vi "MTUChipCornerSample.vi"() -> ()   [LabVIEW 2017, in "AOILib_MTUchipcorner_V1.lvlib"]
uses:
  <userlib>/AOILib_MTUchipcorner_V1/AOILib_MTUchipcorner_V1.lvlib
  <vilib>/vision/NI_Vision_Development_Module.lvlib
panel:
  in  "File Path_IMGin":path=path "C:/Users/MyUser/Desktop/Harvie Test/CornerChip/ChipCornerTest.bmp"
  out "image":T1(plugin-control)
  out "X Resolution":i32
  out "Y Resolution":i32
  in  "imageParm 2":T2={"PICmode"=0, "Outputmode"=0, "cols"=2448, "rows"=2048, "correctTheta"=0.0}
  in  "Param":T3={"Select Mode \n0: Dark\n1: light"=1.0, "Threshold Value"=200.0, "Chip Long Side Size"=25.0, "Chip Long Side Min Tolerance"=0.8, "Chip Long Side Max Tolerance"=1.5, "Chip Short Side Size"=15.0, "Chip Short Side Min Tolerance"=0.8, "Chip Short Side Max Tolerance"=1.5, "Chip Pitch X"=70.0, "Chip Pitch Y"=70.0, "Edge Exclusion Distance"=200.0, "Reserve[11]"=0.0, "Reserve[12]"=0.0, "Parameters[13]"=0.0, "Parameters[14]"=0.0, "Parameters[15]"=0.0, "Parameters[16]"=0.0, "Parameters[17]"=0.0, "Parameters[18]"=0.0, "Parameters[19]"=0.0}
  out "image out":T1(plugin-control)
  out "error out":errorcluster
  out "fAngle":sgl[](array[numeric])
  out "fPosY":sgl[](array[numeric])
  out "fPosX":sgl[](array[numeric])
  out "boolResult":sgl[](array[numeric])
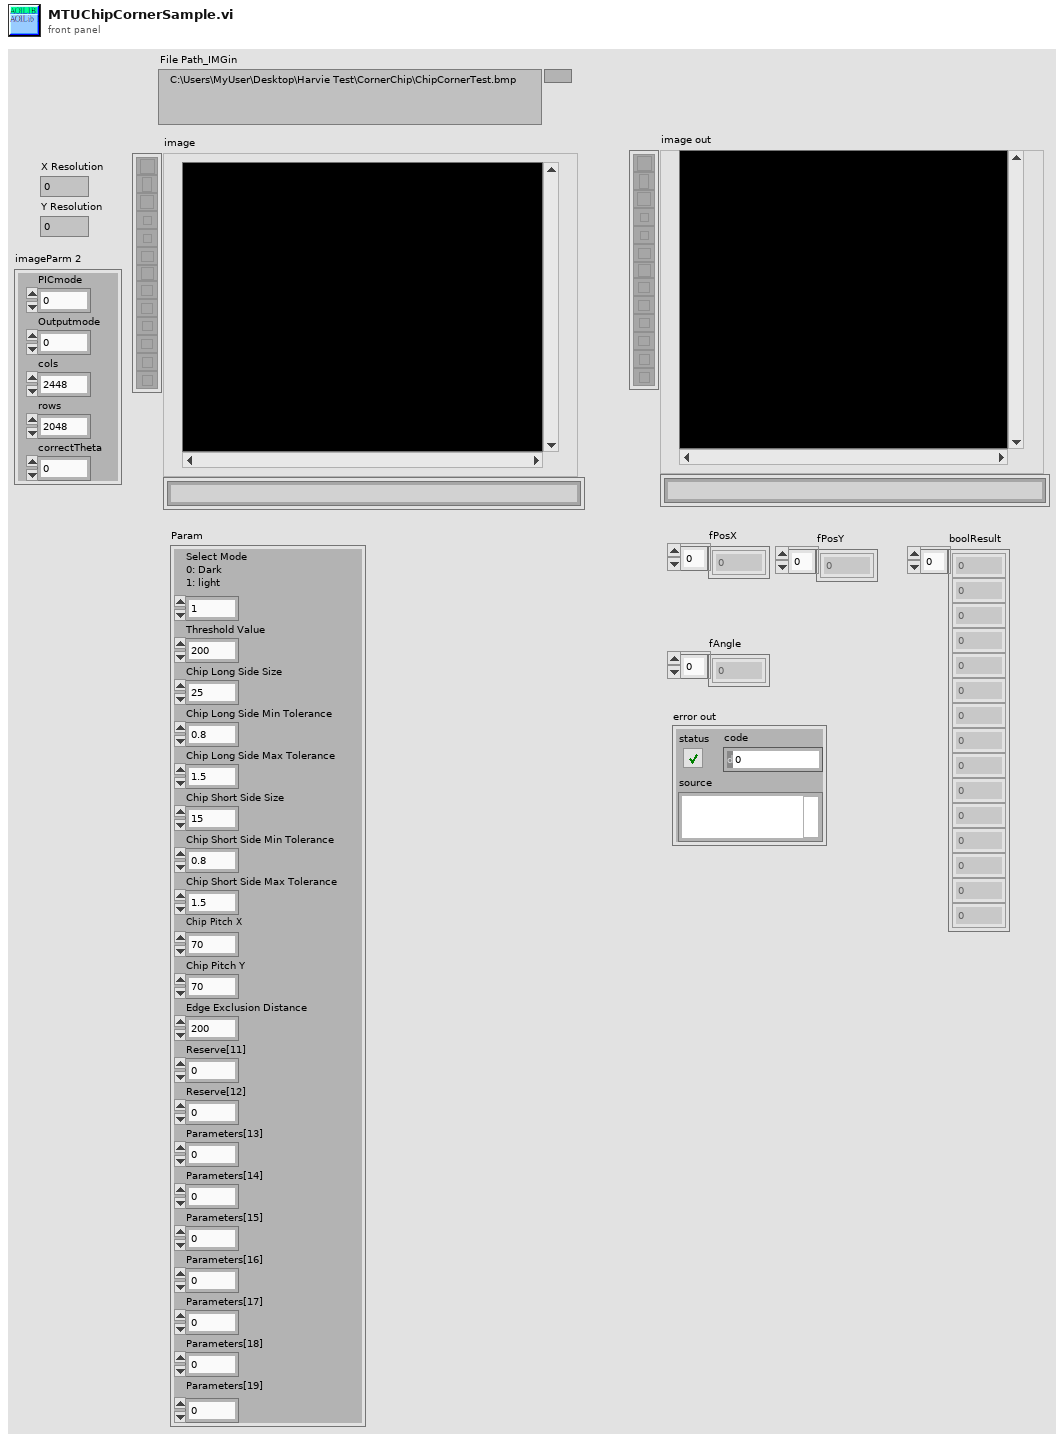
[diagram p1: front panel]
types:
  T1 = typedef "IMAQ Image.ctl" = refnum<image>
  T2 = cluster{"PICmode":i32, "Outputmode":i32, "cols":i32, "rows":i32, "correctTheta":dbl}
  T3 = cluster{"Select Mode \n0: Dark\n1: light":sgl, "Threshold Value":sgl, "Chip Long Side Size":sgl, "Chip Long Side Min Tolerance":sgl, "Chip Long Side Max Tolerance":sgl, "Chip Short Side Size":sgl, "Chip Short Side Min Tolerance":sgl, "Chip Short Side Max Tolerance":sgl, "Chip Pitch X":sgl, "Chip Pitch Y":sgl, "Edge Exclusion Distance":sgl, "Reserve[11]":sgl, "Reserve[12]":sgl, "Parameters[13]":sgl, "Parameters[14]":sgl, "Parameters[15]":sgl, "Parameters[16]":sgl, "Parameters[17]":sgl, "Parameters[18]":sgl, "Parameters[19]":sgl}
  T4 = typedef "Image Type" = u32
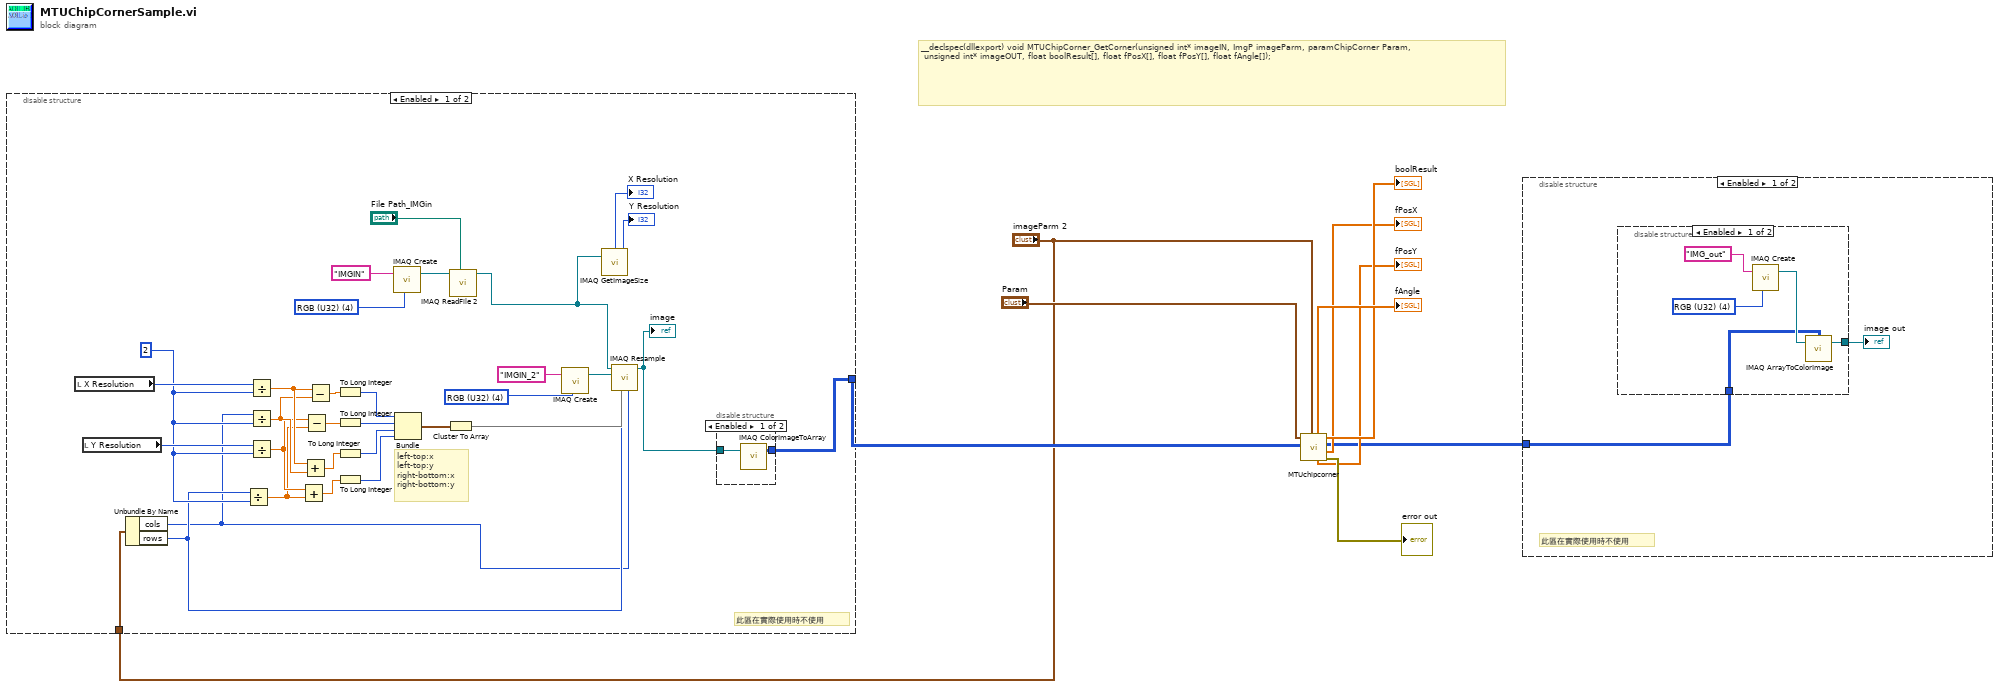
[diagram p0: block diagram]
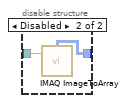
[diagram p2: hidden frame]
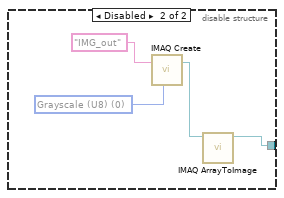
[diagram p4: hidden frame]
diagram:
  # "__declspec(dllexport) void MTUChipCorner_GetCorner(unsigned int* imageIN, ImgP imageParm, paramChipCorner Param,\n\tunsigned int* imageOUT, float boolResult[], float fPosX[], float fPosY[], float fAngle[]);"
  n1 = disable-structure shown="Enabled" {
    disable-tunnel: [w14 _] -> w2
    disable-tunnel: "imageParm 2" -> [w12 _]
    frame Enabled {
      w16 = T4 4 items=["Grayscale (U8)", "Grayscale (I16)", "Grayscale (SGL)", "Complex (CSG)", "RGB (U32)", "HSL (U32)", "RGB (U64)", "Grayscale (U16)"] ("Image Type")
      w17 = T4 4 items=["Grayscale (U8)", "Grayscale (I16)", "Grayscale (SGL)", "Complex (CSG)", "RGB (U32)", "HSL (U32)", "RGB (U64)", "Grayscale (U16)"] ("Image Type")
      w32 = 2 ("y")
      # "此區在實際使用時不使用"
      # "left-top:x\nleft-top:y\nright-bottom:x\nright-bottom:y"
      n2 = local read "X Resolution"() -> (w34:i32)
      n3 = local read "Y Resolution"() -> (w33:i32)
      n4 = Unbundle By Name(w12) -> ("cols"=w10:i32, "rows"=w11:i32)
      n5 = Divide(x=w11, y=w32) -> (x/y=w25:dbl)
      n6 = Divide(x=w34, y=w32) -> (x/y=w29:dbl)
      n7 = Divide(x=w10, y=w32) -> (x/y=w28:dbl)
      n8 = Divide(x=w33, y=w32) -> (x/y=w26:dbl)
      n9 = Add(x=w26, y=w25) -> (x+y=w24:dbl)
      n10 = Add(x=w29, y=w28) -> (x+y=w27:dbl)
      n11 = Subtract(x=w26, y=w25) -> (x-y=w30:dbl)
      n12 = Subtract(x=w29, y=w28) -> (x-y=w31:dbl)
      n13 = To Long Integer(number=w31) -> (32bit integer=w23:i32)
      n14 = To Long Integer(number=w30) -> (32bit integer=w22:i32)
      n15 = To Long Integer(number=w27) -> (32bit integer=w21:i32)
      n16 = To Long Integer(number=w24) -> (32bit integer=w20:i32)
      n17 = call "IMAQ Create"("Image Name"="IMGIN", "Image Type"=w17) -> ("New Image"=w40:T1)  [unwired: 3 in, 1 out]
      n18 = Bundle(w23, w22, w21, w20) -> (w19:cluster{i32, i32, i32, i32})  [unwired: 1 in]
      n19 = Cluster To Array(cluster=w19) -> (array=w18:i32[])
      n20 = call "IMAQ ReadFile 2"("File Path"="File Path_IMGin", "Image"=w40) -> ("Image Out"=w15:T1)  [unwired: 5 in, 4 out]
      n21 = call "IMAQ Create"("Image Name"="IMGIN_2", "Image Type"=w16) -> ("New Image"=w37:T1)  [unwired: 3 in, 1 out]
      n22 = call "IMAQ GetImageSize"("Image"=w15) -> ("Y Resolution"=→"Y Resolution":i32, "X Resolution"=→"X Resolution":i32)  [unwired: 3 in, 1 out]
      n23 = call "IMAQ Resample"("X Resolution"=w10, "Optional Rectangle"=w18, "Y Resolution"=w11, "Image Dst"=w37, "Image Src"=w15) -> ("Image Dst Out"=w13:T1)  [unwired: 5 in, 1 out]
      "image" <- w13
      n24 = disable-structure shown="Enabled" {
        disable-tunnel: w13 -> [w43 w45]
        disable-tunnel: [w42 w44] -> w14
        frame Enabled {
          n25 = call "IMAQ ColorImageToArray"("Image"=w43) -> ("Image Pixels (U32)"=w42:u32[][])  [unwired: 3 in, 2 out]
        }
        frame Disabled {
          n26 = call "IMAQ ImageToArray"("Image"=w45) -> ("Image Pixels (U8)"=w44:u8[][])  [unwired: 3 in, 4 out]
        }
      }
    }
    frame Disabled {
    }
  }
  n27 = call <userlib>:"MTUchipcorner.vi"("imageParm in"="imageParm 2", "Image Pixels (U32)"=w2, "Param"="Param") -> ("error out"=→"error out":errorcluster, "fPosX"=→"fPosX":sgl[], "imageOUT"=w4:u32[][], "boolResult"=→"boolResult":sgl[], "fPosY"=→"fPosY":sgl[], "fAngle"=→"fAngle":sgl[])  [unwired: 3 in]
  n28 = disable-structure shown="Enabled" {
    disable-tunnel: w4 -> [w46 _]
    frame Enabled {
      # "此區在實際使用時不使用"
      n29 = disable-structure shown="Enabled" {
        disable-tunnel: [w51 w56] -> w47
        disable-tunnel: w46 -> [w48 _]
        frame Enabled {
          w49 = T4 4 items=["Grayscale (U8)", "Grayscale (I16)", "Grayscale (SGL)", "Complex (CSG)", "RGB (U32)", "HSL (U32)", "RGB (U64)", "Grayscale (U16)"] ("Image Type")
          n30 = call "IMAQ Create"("Image Name"="IMG_out", "Image Type"=w49) -> ("New Image"=w52:T1)  [unwired: 3 in, 1 out]
          n31 = call "IMAQ ArrayToColorImage"("Image Pixels (U32)"=w48, "Image"=w52) -> ("Image Out"=w51:T1)  [unwired: 3 in, 1 out]
        }
        frame Disabled {
          w57 = T4 0 items=["Grayscale (U8)", "Grayscale (I16)", "Grayscale (SGL)", "Complex (CSG)", "RGB (U32)", "HSL (U32)", "RGB (U64)", "Grayscale (U16)"] ("Image Type")
          n32 = call "IMAQ Create"("Image Name"="IMG_out", "Image Type"=w57) -> ("New Image"=w53:T1)  [unwired: 3 in, 1 out]
          n33 = call "IMAQ ArrayToImage"("Image"=w53) -> ("Image Out"=w56:T1, "Image Pixels (U8)"=w55:u8[][])  [unwired: 8 in, 1 out]
        }
      }
      "image out" <- w47
    }
    frame Disabled {
    }
  }
